vi "Exercise1.7-Read wav and Play.vi"() -> ()   [LabVIEW 2013]
uses:
  <vilib>/sound2/lvsound2.llb/Sound File Info (path).vi
  <vilib>/sound2/lvsound2.llb/Sound File Read Open.vi
  <vilib>/sound2/lvsound2.llb/Sound File Read (DBL).vi
panel:
  in  "Read path":path
  in  "Save path":path
  out "Waveform":waveform(dbl)
  out "Waveform array":waveform(dbl)[](array[waveform])
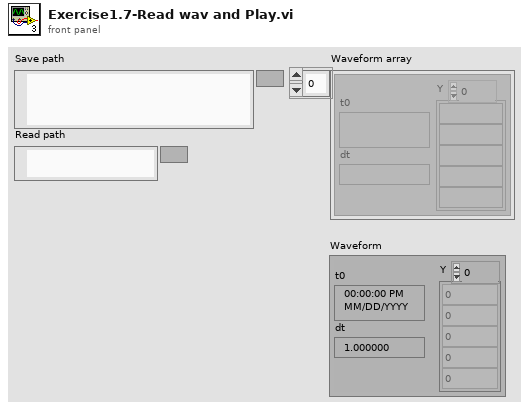
[diagram p1: front panel]
types:
  T1 = typedef "Sound File Refnum.ctl" = refnum<file>
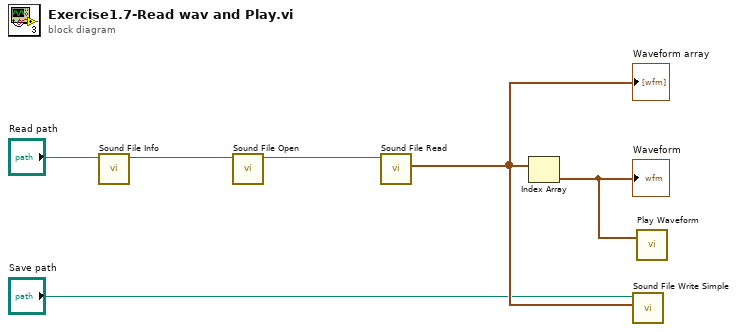
[diagram p0: block diagram]
diagram:
  n1 = call-poly <vilib>:"Sound File Info.vi"("path"="Read path") -> ("path out"=w6:path)  [unwired: 7 in, 3 out]
  n2 = call-poly <vilib>:"Sound File Open.vi"("path"=w6) -> ("sound file refnum"=w5:T1)  [unwired: 9 in, 1 out]
  n3 = call-poly <vilib>:"Sound File Read.vi"("sound file refnum"=w5) -> ("data"=w4:waveform(dbl)[])  [unwired: 6 in, 4 out]
  "Waveform array" <- w4
  n4 = Index Array "Index Array"(array=w4) -> (element=w3:waveform(dbl))  [unwired: 1 in]
  "Waveform" <- w3
  n5 = call <vilib>:"Sound File Write Simple.vi"("data"=w4, "path"="Save path") -> ()  [unwired: 8 in, 2 out]
  n6 = call "Play Waveform"("Data"=w3) -> ()  [unwired: 18 in, 1 out]
